vi "Memory.Pointer.Write.Safe.1D.I64.vi"(8 "error in (no error)":errorcluster, 9 "count":u64 format="%d elements", 10 "buffer in":i64[](array[numeric]), 11 "pointer in":refnum<class "Memory.Pointer.lvclass">) -> (0 "error out":errorcluster, 1 "count out":u64 format="%d elements", 2 "buffer out":i64[](array[numeric]), 3 "pointer out":refnum<class "Memory.Pointer.lvclass">)   [LabVIEW 2016, in "Memory Manager.lvlib" / "Memory.Pointer.lvclass"]
doc: "Writes <b>count</b> elements from the provided <b>buffer</b> to the address specified by <b>pointer</b>.\n\n<b>Note:</b> This VI is <b>safe</b>.\n\nSafe means that this function evaluates the size parameter of <b>pointer</b> to ensure that is inbounds of allocated memory before peforming a memory read/write. Reading/writing more data to a pointer than it has allocated can corrupt or crash LabVIEW."
uses:
  Memory.Pointer.lvclass
  Memory.Pointer.lvclass/Memory.Pointer.ctl
  Accessors/Get Address.vi
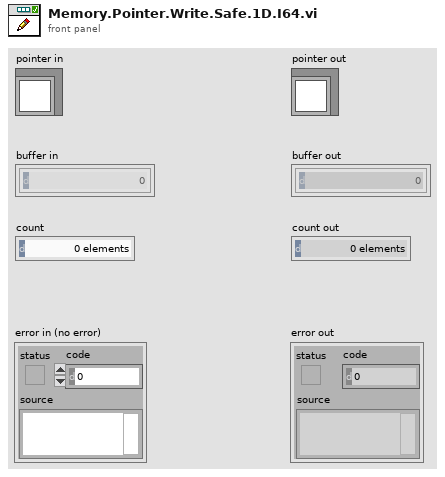
[diagram p1: front panel]
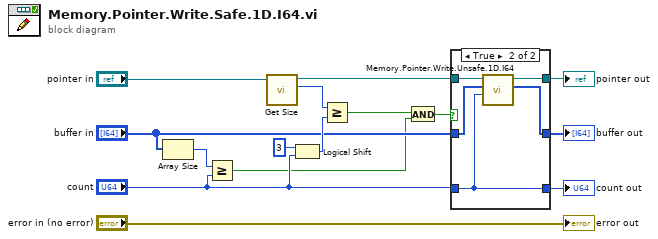
[diagram p0: block diagram]
diagram:
  n1 = Array Size(array="buffer in") -> (size(s)=w4:i32)
  n2 = Greater Or Equal?(x=w4, y="count") -> (x >= y?=w2:bool)
  n3 = call "Get Size.vi"("Pointer in"="pointer in") -> ("size"=w12:u64, "Pointer out"=w11:refnum<class "Memory.Pointer.lvclass">)  [unwired: 8 in, 1 out]
  n4 = Logical Shift(y=i16 3, x="count") -> (x << y=w13:u64)
  n5 = Greater Or Equal?(x=w12, y=w13) -> (x >= y?=w6:bool)
  n6 = And(x=w6, y=w2) -> (x .and. y?=w7:bool)
  n7 = case shown="True" w7 {
    tunnel: w11 -> [w18 w23]
    tunnel: [w18 w22] -> w10
    tunnel: [w17 w21] -> w9
    tunnel: "count" -> [w16 w19]
    tunnel: "buffer in" -> [w17 w20]
    tunnel: [w16 w19] -> w1
    frame False {
    }
    frame True {
      n8 = call "Memory.Pointer.Write.Unsafe.1D.I64.vi"("count"=w19, "buffer in"=w20, "pointer in"=w23) -> ("buffer out"=w21:i64[], "pointer out"=w22:refnum<class "Memory.Pointer.lvclass">)  [unwired: 5 in, 2 out]
    }
  }
  "pointer out" <- w10
  "buffer out" <- w9
  "count out" <- w1
  "error out" <- "error in (no error)"
